vi "Send Value to Datalogger.vi"(8 "error in (no error)":errorcluster, 10 "Data Record":T1, 11 "MWWL Verification in":refnum<class "MWWL Verification.lvclass">) -> (0 "error out":errorcluster, 3 "MWWL Verification out":refnum<class "MWWL Verification.lvclass">)   [LabVIEW 2018, in "MWWL Verification.lvlib" / "MWWL Verification.lvclass"]
uses:
  MWWL Verification.lvclass
  Type Defs/Data Record Control.ctl
  MWWL Verification.lvclass/MWWL Verification.ctl
  Datalogger Actor/Datalogger Actor Messages/Log Value to File Msg/Log Value to File Msg.lvclass/Log Value to File Msg.ctl
  <vilib>/ActorFramework/Message Enqueuer/Message Enqueuer.lvclass/Message Enqueuer.ctl
  <vilib>/ActorFramework/Message Enqueuer/Enqueue.vi
  <vilib>/ActorFramework/Message Enqueuer/Init from Existing Queue.vi
  Datalogger Actor/Datalogger Actor Messages/Log Value to File Msg/Log Value to File Msg.lvclass
  C:/Program Files (x86)/National Instruments/LabVIEW 2018/vi.lib/ActorFramework/Message/Message.lvclass
  <vilib>/ActorFramework/Message Priority Queue/Priority Enqueue.vi
  <vilib>/ActorFramework/Message Enqueuer/Message Enqueuer.lvclass
  <vilib>/ActorFramework/Actor/Actor.lvclass
  C:/Program Files (x86)/National Instruments/LabVIEW 2018/vi.lib/ActorFramework/Actor/Actor.lvclass
  MWWL Verification.lvlib
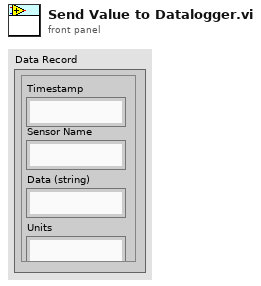
[diagram p1: front panel]
types:
  T1 = typedef "MWWL Verification.lvlib/Data Record Control.ctl" = cluster{"Timestamp":string, "Sensor Name":string, "Data (string)":string, "Units":string}
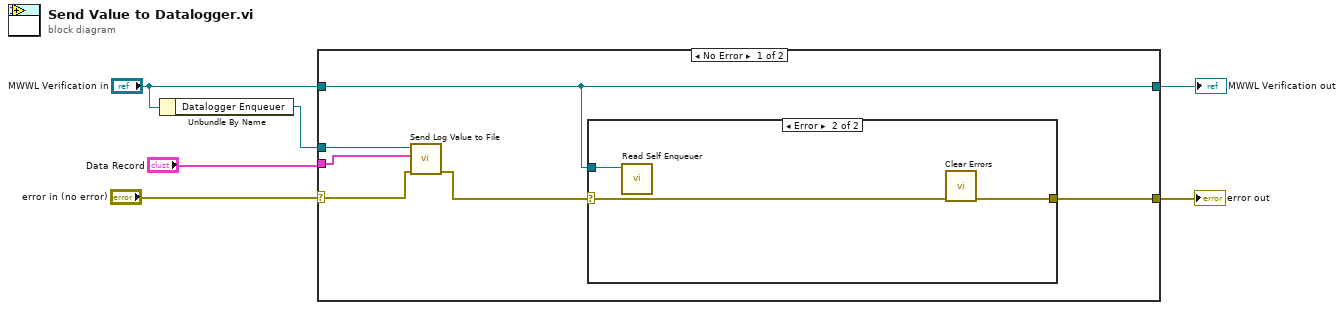
[diagram p0: block diagram]
diagram:
  n1 = Unbundle By Name("MWWL Verification in") -> ("Datalogger Enqueuer"=w2:refnum<class "Message Enqueuer.lvclass">)
  n2 = case shown="No Error" "error in (no error)" {
    selector: "error in (no error)" -> [w9 w18]
    tunnel: [w12 w18] -> w5
    tunnel: [w7 w17] -> w4
    tunnel: "MWWL Verification in" -> [w7 w17]
    tunnel: "Data Record" -> [w10 _]
    tunnel: w2 -> [w11 _]
    frame No Error {
      n3 = call "Send Log Value to File.vi"("error in (no error)"=w9, "Data Record"=w10, "Message Enqueuer in"=w11) -> ("error out"=w8:errorcluster)  [unwired: 7 in, 1 out]
      n4 = case shown="Error" w8 {
        selector: w8 -> [w13 w14]
        tunnel: [w13 w15] -> w12
        tunnel: w7 -> [_ w16]
        frame No Error {
        }
        frame Error {
          n5 = call <vilib>:"Read Self Enqueuer.vi"("Actor"=w16) -> ()  [unwired: 10 in, 1 out]
          n6 = call <vilib>:"Clear Errors.vi"("error in (no error)"=w14) -> ("error out"=w15:errorcluster)  [unwired: 5 in, 1 out]
        }
      }
    }
    frame Error {
    }
  }
  "error out" <- w5
  "MWWL Verification out" <- w4
